vi "登录界面.vi"() -> ()   [LabVIEW 2013]
panel:
  in  "取消按钮":bool
  out "error out":errorcluster caption="错误输出"
  in  "用户登陆":bool
  in  "用户密码":string
  in  "用户名称":string(combo)
  # "***电器信息化"
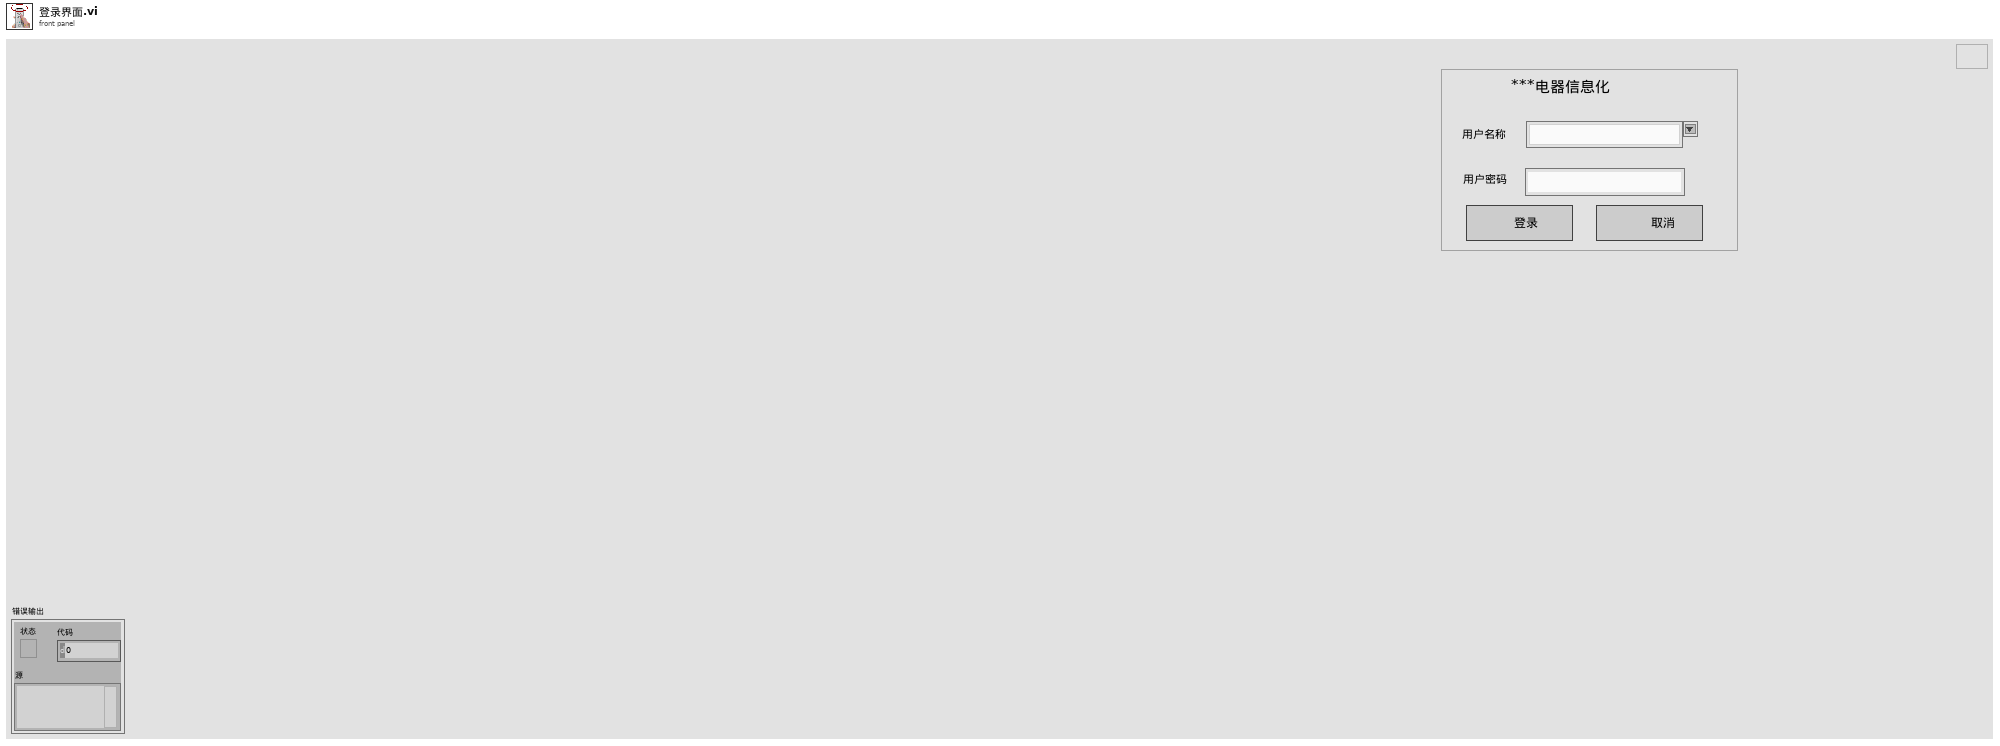
[diagram p1: front panel]
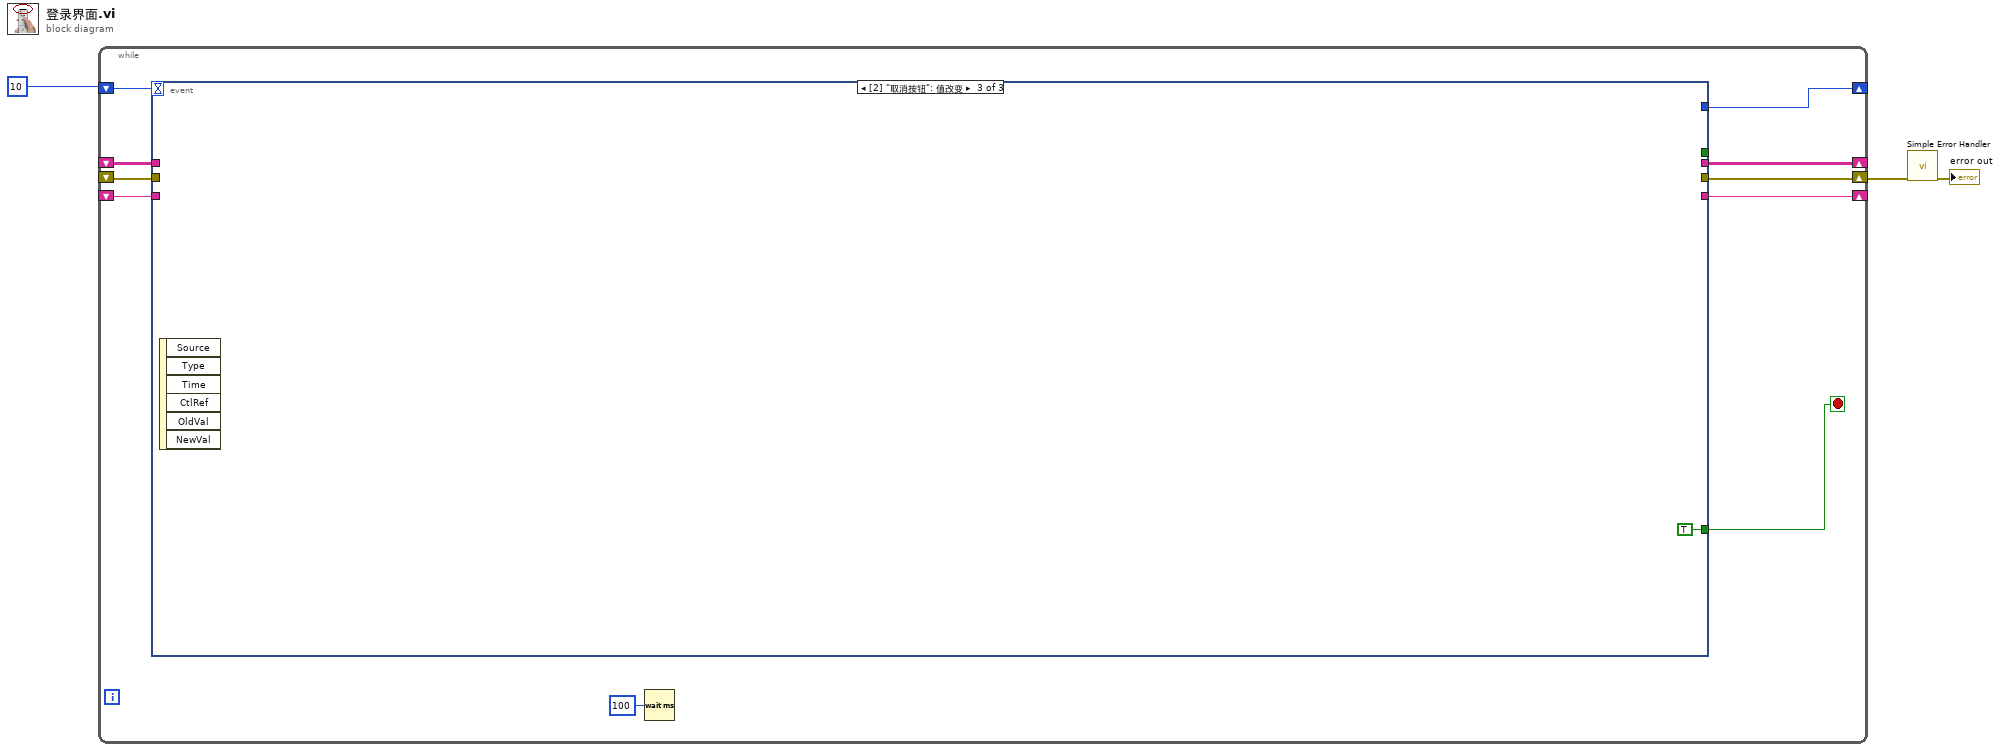
[diagram p0: block diagram]
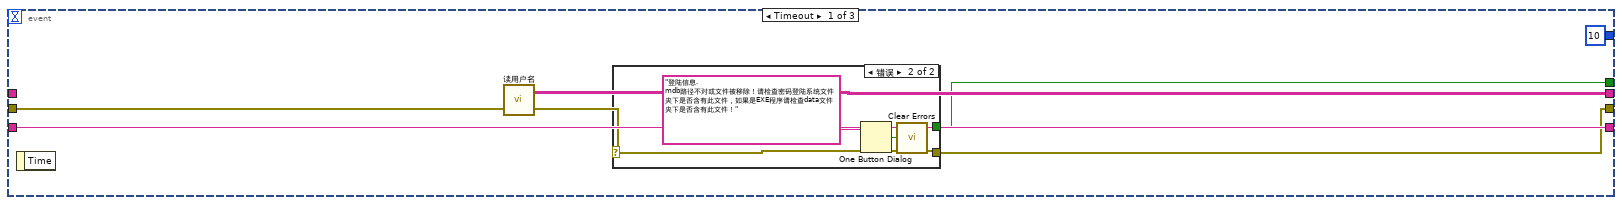
[diagram p2: hidden frame]
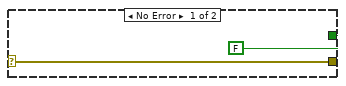
[diagram p3: hidden frame]
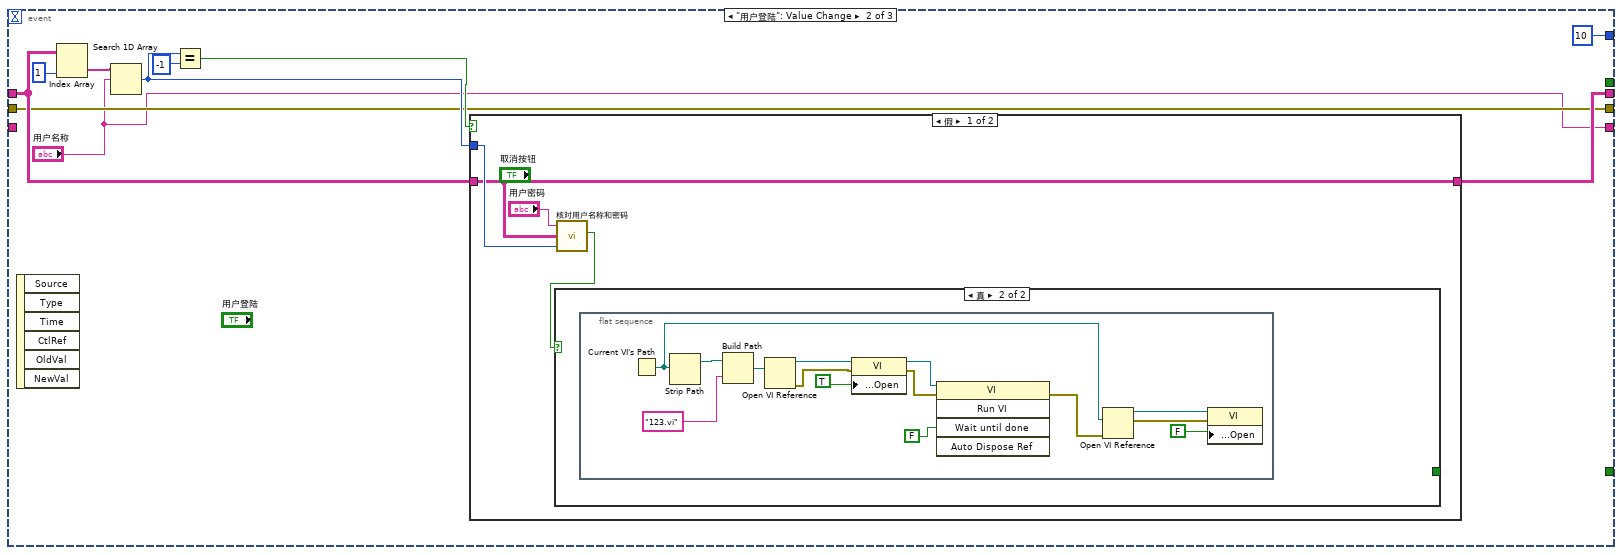
[diagram p4: hidden frame]
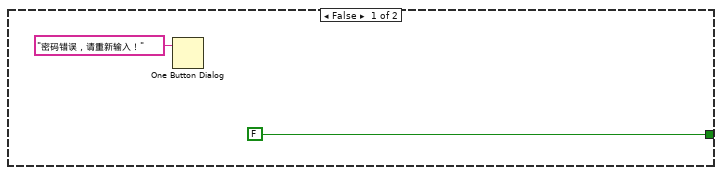
[diagram p5: hidden frame]
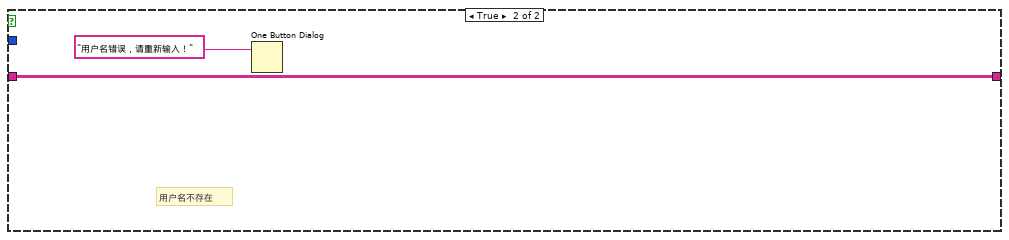
[diagram p6: hidden frame]
diagram:
  n1 = while {
    shift-right: [w6] -> _
    shift-left: _ -> [w10]
    shift-right: [w13] -> w2
    shift-left: _ -> [w9]
    shift-right: [w11] -> _
    shift-left: 10 -> [w12]
    shift-right: [w8] -> _
    shift-left: _ -> [w7]
    stop <- w4 stop-if-true
    n2 = event shown="[2] \"取消按钮\": 值改变" {
      selector: _ -> [_ _ _]
      dyn-events: _ -> [_ _ _]
      timeout: w12 -> [_ _ _]
      tunnel: [w18 w30 _] -> w6
      tunnel: [w16 w29 _] -> w13
      tunnel: [10 10 _] -> w11
      tunnel: w10 -> [_ w32 _]
      tunnel: w9 -> [w14 w29 _]
      tunnel: [w19 "用户名称" _] -> w8
      tunnel: w7 -> [w19 _ _]
      tunnel: [w15 _ _] -> _
      tunnel: [_ _ TRUE] -> w4
      event Timeout {
        n3 = event-data() -> ()  [unwired: 2 out]
        n4 = call "读用户名.vi"("error in (no error)"=w14) -> ("error out"=w17:errorcluster, "SQL Results"=w18:string[][])  [unwired: 1 in]
        n5 = case shown="错误" w17 {
          selector: w17 -> [w22 w26]
          tunnel: [w22 w25] -> w16
          tunnel: [FALSE ("true") w23] -> w15
          frame No Error {
          }
          frame Error {
            n6 = One Button Dialog(message="登陆信息.mdb路径不对或文件被移除！请检查密码登陆系统文件夹下是否含有此文件，如果是EXE程序请检查data文件夹下是否含有此文件！" ("消息")) -> (true=w23:bool)  [unwired: 1 out]
            n7 = call <vilib>:"Clear Errors.vi"("error in (no error)"=w26) -> ("error out"=w25:errorcluster)  [unwired: 6 out]
          }
        }
      }
      event "用户登陆": Value Change {
        n8 = event-data() -> ()  [unwired: 7 out]
        n9 = Index Array(array=w32, index (col)=1 ("禁用的索引 (列)")) -> (element=w28:string[])  [unwired: 1 in]
        n10 = Search 1D Array(1D array=w28, element="用户名称") -> (index of element=w31:i32)  [unwired: 1 out]
        n11 = Equal?(x=w31, y=-1) -> (x = y?=w34:bool)
        n12 = case shown="假" w34 {
          tunnel: w32 -> [w38 w57]
          tunnel: w31 -> [w40 _]
          tunnel: [w38 w57] -> w30
          frame False {
            n13 = call "核对用户名称和密码.vi"("用户密码"="用户密码", "Data"=w38, "index of element"=w40) -> ("布尔"=w39:bool)  [unwired: 3 out]
            n14 = case shown="真" w39 {
              tunnel: [FALSE _] -> _
              frame False {
                n15 = One Button Dialog(message="密码错误，请重新输入！" ("消息")) -> ()  [unwired: 2 out]
              }
              frame True {
                n16 = flat-sequence {
                  frame #0 {
                    n17 = Current VI's Path() -> (path=w45:path)
                    n18 = Strip Path(path=w45) -> (stripped path=w56:path)  [unwired: 1 out]
                    n19 = Build Path(base path=w56, name or relative path="123.vi" ("名称或相对路径")) -> (appended path=w55:path)
                    n20 = Open VI Reference(vi path=w55) -> (vi reference=w54:refnum<vi>, error out=w53:errorcluster)  [unwired: 5 in]
                    n21 = property on="Property Node" class="VI"(reference=w54, error in=w53, "Front Panel Window:Open"=TRUE) -> (reference out=w44:refnum<vi>, error out=w43:errorcluster)
                    n22 = invoke class="VI" method="Run VI"(reference=w44, error in=w43, "Wait until done"=FALSE) -> (error out=w46:errorcluster)  [unwired: 2 in, 4 out]
                    n23 = Open VI Reference(vi path=w45, error in (no error)=w46) -> (vi reference=w50:refnum<vi>, error out=w48:errorcluster)  [unwired: 4 in]
                    n24 = property on="Property Node" class="VI"(reference=w50, error in=w48, "Front Panel Window:Open"=FALSE) -> ()  [unwired: 2 out]
                  }
                }
              }
            }
          }
          frame True {
            # "用户名不存在"
            n25 = One Button Dialog(message="用户名错误，请重新输入！" ("消息")) -> ()  [unwired: 2 out]
          }
        }
      }
      event "取消按钮": Value Change {
        n26 = event-data() -> ()  [unwired: 7 out]
      }
    }
    n27 = Wait (ms)(milliseconds to wait=u32 100 ("等待时间（毫秒）")) -> ()  [unwired: 1 out]
  }
  n28 = call <vilib>:"Simple Error Handler.vi"("error in (no error)"=w2) -> ("error out"=→"error out":errorcluster)  [unwired: 1 in, 7 out]
